vi "Async.Close.vi"(8 "error in (no error)":errorcluster, 11 "Async in":refnum<class "VS Inline Async API.lvclass">) -> (0 "error out":errorcluster, 3 "Async out":refnum<class "VS Inline Async API.lvclass">)   [LabVIEW 2015, in "VS Inline Async API.lvlib" / "VS Inline Async API.lvclass"]
uses:
  VS Inline Async API.lvclass
  VS Inline Async API.lvclass/VS Inline Async API.ctl
  <vilib>/NI Veristand/Custom Device Tools/Custom Device Utility Library/NI VeriStand - Print Debug String.vi
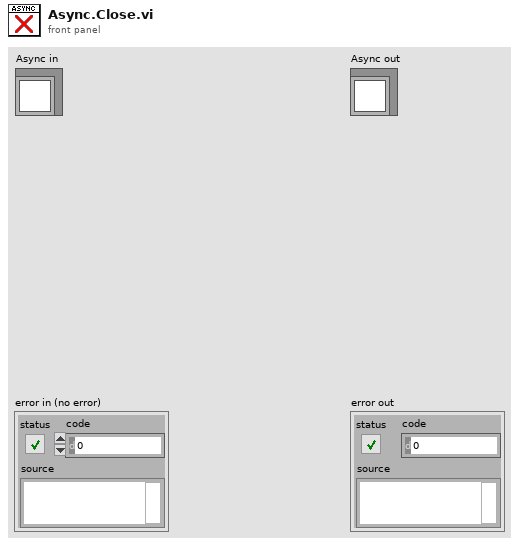
[diagram p1: front panel]
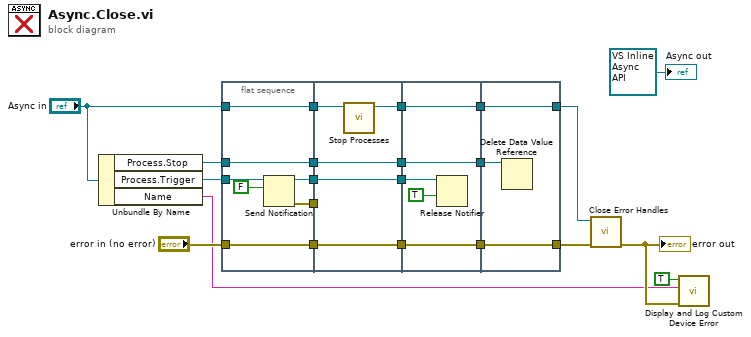
[diagram p0: block diagram]
diagram:
  n1 = Unbundle By Name("Async in") -> ("Process.Stop"=w8:refnum<data-value>, "Process.Trigger"=w15:refnum<notifier>, "Name"=w11:string)
  n2 = flat-sequence {
    tunnel: [w29] -> w22
    tunnel: "error in (no error)" -> [w29]
    tunnel: [w27] -> w18
    tunnel: [w26] -> w16
    tunnel: w15 -> [w25]
    tunnel: [w24] -> w10
    tunnel: "Async in" -> [w24]
    tunnel: w8 -> [w23]
    tunnel: [w23] -> w5
    tunnel: [w34] -> w21
    tunnel: w22 -> [w34]
    tunnel: w18 -> [_]
    tunnel: [w33] -> w17
    tunnel: w16 -> [w33]
    tunnel: w10 -> [w32]
    tunnel: [w31] -> w6
    tunnel: w5 -> [w31]
    tunnel: [w30] -> w3
    tunnel: w21 -> [w39]
    tunnel: w17 -> [w37]
    tunnel: [w39] -> w9
    tunnel: [w36] -> w7
    tunnel: w6 -> [w36]
    tunnel: [w35] -> w4
    tunnel: w3 -> [w35]
    tunnel: [w42] -> w19
    tunnel: w9 -> [w42]
    tunnel: w7 -> [w41]
    tunnel: [w40] -> w1
    tunnel: w4 -> [w40]
    frame #0 {
      n3 = Send Notification(notification=FALSE, notifier=w25) -> (notifier out=w26:refnum<notifier>, error out=w27:errorcluster)  [unwired: 1 in]
    }
    frame #1 {
      n4 = call "Stop Processes.vi"("VS Inline Async API in"=w32) -> ("VS Inline Async API out"=w30:refnum<class "VS Inline Async API.lvclass">)  [unwired: 10 in]
    }
    frame #2 {
      n5 = Release Notifier(notifier=w37, force destroy? (F)=TRUE ("notification")) -> ()  [unwired: 1 in, 3 out]
    }
    frame #3 {
      n6 = Delete Data Value Reference(data value reference=w41) -> ()  [unwired: 1 in, 2 out]
    }
  }
  n7 = call "Close Error Handles.vi"("error in"=w19, "Async in"=w1) -> ("error out"=w13:errorcluster)  [unwired: 8 in, 1 out]
  "error out" <- w13
  n8 = call "Display and Log Custom Device Error.vi"("error out"=w13, "Your code's public name"=w11, "Custom Device? (T)"=TRUE) -> ()  [unwired: 9 in]
  "Async out" <- refnum<class "VS Inline Async API.lvclass"> refnum ("Async out")
